vi "test_Add Custom Device.vi"(8 "error in (no error)":errorcluster, 11 "TestCase in":refnum<class "Scan Engine Unit Tests.lvclass">) -> (0 "error out":errorcluster, 3 "TestCase out":refnum<class "Scan Engine Unit Tests.lvclass">)   [LabVIEW 2017, in "Scan Engine Scripting API Custom Device Unit Tests.lvclass"]
uses:
  Scan Engine Scripting API Custom Device Unit Tests.lvclass
  Scan Engine Unit Tests.lvclass
  Type Defs/Main Settings.ctl
  <vilib>/addons/_JKI Toolkits/VI Tester/TestCase.llb/TestCase.lvclass
  Scripting/Scan Engine Scripting.lvlib
  Scan Engine Custom Device.lvlib
  C:/Program Files (x86)/National Instruments/LabVIEW 2017/vi.lib/addons/_JKI Toolkits/VI Tester/TestCase.llb/TestCase.lvclass
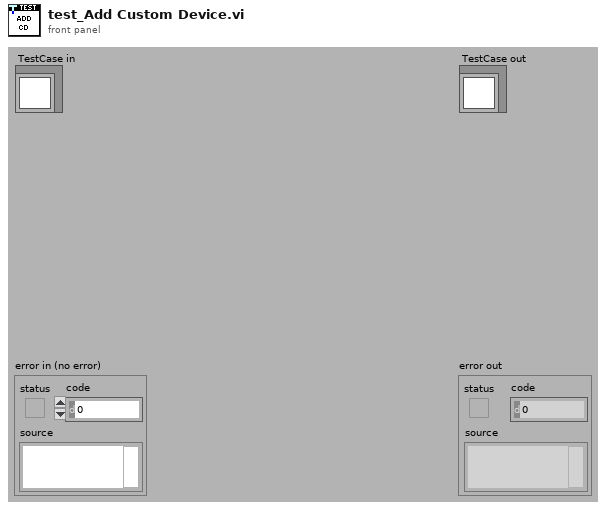
[diagram p1: front panel]
types:
  T1 = typedef "Scan Engine Custom Device.lvlib/Main Settings.ctl" = cluster{"sync to scan":bool, "scan engine decimation":u16, "delay after FPGA load (s)":u16}
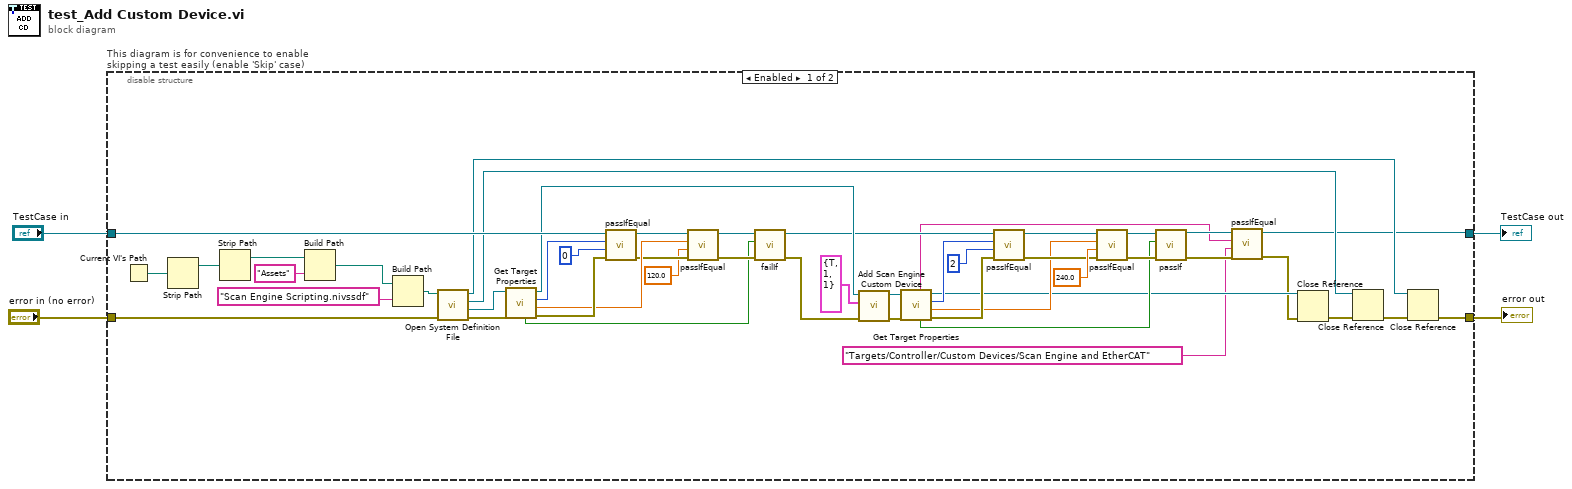
[diagram p0: block diagram]
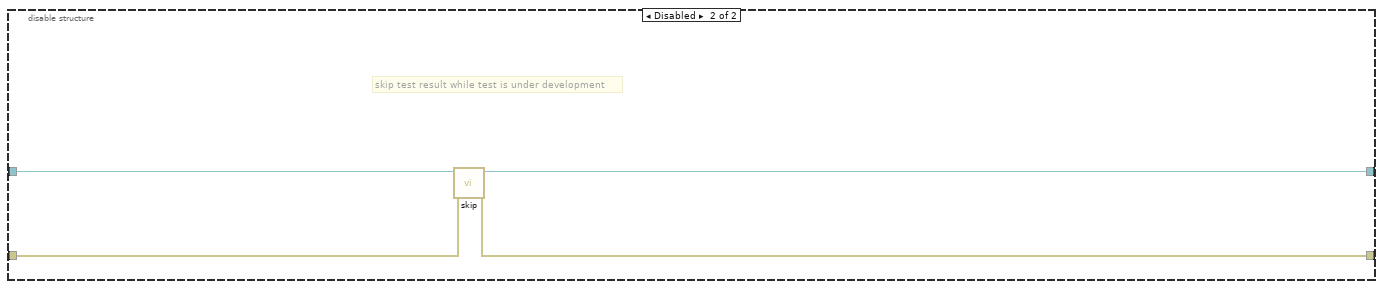
[diagram p2: hidden frame]
diagram:
  n1 = disable-structure "This diagram is for convenience to enable skipping a test easily (enable 'Skip' case)" shown="Enabled" {
    disable-tunnel: "TestCase in" -> [w42 w57]
    disable-tunnel: [w7 w55] -> w1
    disable-tunnel: [w12 w56] -> w3
    disable-tunnel: "error in (no error)" -> [w46 w54]
    frame Enabled {
      n2 = Current VI's Path() -> (path=w53:path)
      n3 = Strip Path(path=w53) -> (stripped path=w52:path)  [unwired: 1 out]
      n4 = Strip Path(path=w52) -> (stripped path=w51:path)  [unwired: 1 out]
      n5 = Build Path(base path=w51, name or relative path="Assets") -> (appended path=w49:path)
      n6 = Build Path(base path=w49, name or relative path="Scan Engine Scripting.nivssdf") -> (appended path=w47:path)
      n7 = call "Open System Definition File.vi"("error in"=w46, "path"=w47) -> ("error out"=w43:errorcluster, "target ref"=w44:refnum<k24>, "root ref"=w16:refnum<k24>, "system definition ref"=w13:refnum<k24>)  [unwired: 6 in]
      n8 = call "Get Target Properties.vi"("error in"=w43, "target ref in"=w44) -> ("error out"=w39:errorcluster, "TL timeout value"=w38:dbl, "ts value"=w41:u32, "target ref out"=w31:refnum<k24>, "dependent node found"=w5:bool)  [unwired: 4 in, 1 out]
      n9 = call-dynamic "passIfEqual.vi"("error in (no error)"=w39, "y"=u32 0 ("ts value"), "x"=w41, "TestCase in"=w42) -> ("error out"=w36:errorcluster, "TestCase out"=w37:refnum<class "Scan Engine Unit Tests.lvclass">)  [unwired: 6 in]
      n10 = call-dynamic "passIfEqual.vi"("error in (no error)"=w36, "y"=120.0 ("TL timeout value"), "x"=w38, "TestCase in"=w37) -> ("error out"=w34:errorcluster, "TestCase out"=w33:refnum<class "Scan Engine Unit Tests.lvclass">)  [unwired: 6 in]
      n11 = call-dynamic "failIf.vi"("error in (no error)"=w34, "fail"=w5, "TestCase in"=w33) -> ("error out"=w32:errorcluster, "TestCase out"=w20:refnum<class "Scan Engine Unit Tests.lvclass">)  [unwired: 7 in]
      n12 = call "Add Scan Engine Custom Device.vi"("error in"=w32, "settings"=T1 {"sync to scan"=TRUE, "scan engine decimation"=1, "delay after FPGA load (s)"=1}, "target in"=w31) -> ("error out"=w24:errorcluster, "target out"=w23:refnum<k24>)  [unwired: 6 in, 1 out]
      n13 = call "Get Target Properties.vi"("error in"=w24, "target ref in"=w23) -> ("error out"=w22:errorcluster, "TL timeout value"=w19:dbl, "ts value"=w21:u32, "target ref out"=w17:refnum<k24>, "dependent node found"=w18:bool, "dependent custom device node path"=w9:string)  [unwired: 4 in]
      n14 = call-dynamic "passIfEqual.vi"("error in (no error)"=w22, "y"=u32 2 ("ts value"), "x"=w21, "TestCase in"=w20) -> ("error out"=w27:errorcluster, "TestCase out"=w26:refnum<class "Scan Engine Unit Tests.lvclass">)  [unwired: 6 in]
      n15 = call-dynamic "passIfEqual.vi"("error in (no error)"=w27, "y"=240.0 ("TL timeout value"), "x"=w19, "TestCase in"=w26) -> ("error out"=w29:errorcluster, "TestCase out"=w30:refnum<class "Scan Engine Unit Tests.lvclass">)  [unwired: 6 in]
      n16 = call-dynamic "passIf.vi"("error in (no error)"=w29, "pass"=w18, "TestCase in"=w30) -> ("error out"=w11:errorcluster, "TestCase out"=w10:refnum<class "Scan Engine Unit Tests.lvclass">)  [unwired: 7 in]
      n17 = call-dynamic "passIfEqual.vi"("error in (no error)"=w11, "y"="Targets/Controller/Custom Devices/Scan Engine and EtherCAT", "x"=w9, "TestCase in"=w10) -> ("error out"=w6:errorcluster, "TestCase out"=w7:refnum<class "Scan Engine Unit Tests.lvclass">)  [unwired: 6 in]
      n18 = Close Reference(reference=w17, error in (no error)=w6) -> (error out=w15:errorcluster)
      n19 = Close Reference(reference=w16, error in (no error)=w15) -> (error out=w14:errorcluster)
      n20 = Close Reference(reference=w13, error in (no error)=w14) -> (error out=w12:errorcluster)
    }
    frame Disabled {
      # "skip test result while test is under development"
      n21 = call <vilib>:"skip.vi"("error in (no error)"=w54, "TestCase in"=w57) -> ("error out"=w56:errorcluster, "TestCase out"=w55:refnum<class "Scan Engine Unit Tests.lvclass">)  [unwired: 8 in]
    }
  }
  "error out" <- w3
  "TestCase out" <- w1
